vi "Run TCS.vi"(8 "error in (no error)":errorcluster, 11 "AutoExp in":refnum<class "AutoExp.lvclass">) -> (0 "error out":errorcluster, 3 "AutoExp out":refnum<class "AutoExp.lvclass">)   [LabVIEW 2018, in "AutoExp.lvclass"]
uses:
  AutoExp.lvclass
  AutoExp.lvclass/AutoExp.ctl
  State Machine/State Machine.lvclass
  TCS/TCS.lvclass
  Channel/Channel.lvclass
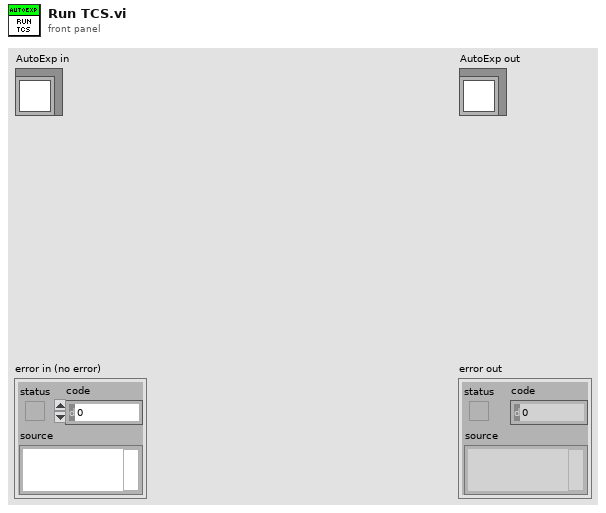
[diagram p1: front panel]
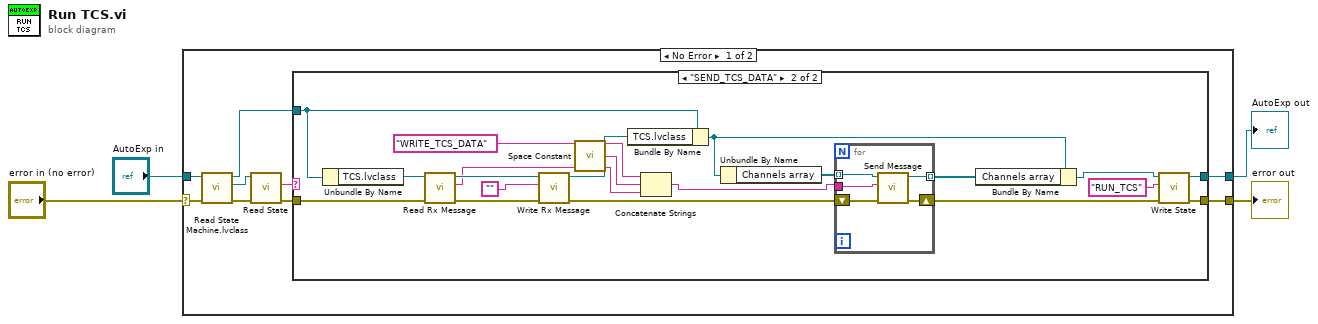
[diagram p0: block diagram]
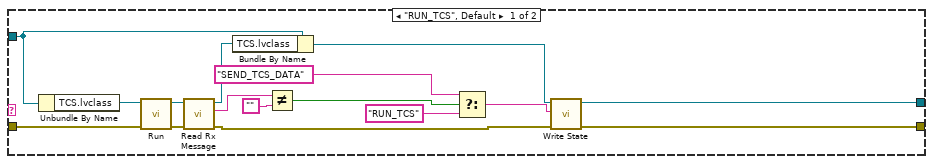
[diagram p2: hidden frame]
diagram:
  n1 = case shown="No Error" "error in (no error)" {
    selector: "error in (no error)" -> [w8 w56]
    tunnel: [w13 w56] -> w3
    tunnel: [w5 w55] -> w1
    tunnel: "AutoExp in" -> [w10 w55]
    frame No Error {
      n2 = call "Read State Machine.lvclass.vi"("error in (no error)"=w8, "AutoExp in"=w10) -> ("error out"=w9:errorcluster, "State Machine.lvclass"=w12:refnum<class "State Machine.lvclass">, "AutoExp out"=w11:refnum<class "AutoExp.lvclass">)  [unwired: 7 in]
      n3 = call-dynamic "Read State.vi"("error in (no error)"=w9, "State Machine in"=w12) -> ("error out"=w6:errorcluster, "State"=w7:string)  [unwired: 7 in, 1 out]
      n4 = case shown="\"SEND_TCS_DATA\"" w7 {
        tunnel: [w25 w36] -> w13
        tunnel: w11 -> [w29 w33]
        tunnel: w6 -> [w14 w34]
        tunnel: [w26 w31] -> w5
        frame "RUN_TCS", Default {
          n5 = Unbundle By Name(w29) -> ("TCS.lvclass"=w17:refnum<class "TCS.lvclass">)
          n6 = call "Run.vi"("error in (no error)"=w14, "TCS in"=w17) -> ("error out"=w15:errorcluster, "TCS out"=w16:refnum<class "TCS.lvclass">)  [unwired: 8 in]
          n7 = call "Read Rx Message.vi"("error in (no error)"=w15, "TCS in"=w16) -> ("error out"=w24:errorcluster, "Rx message"=w23:string, "TCS out"=w28:refnum<class "TCS.lvclass">)  [unwired: 7 in]
          n8 = Bundle By Name(cluster=w29, "TCS.lvclass"=w28) -> (w27:refnum<class "AutoExp.lvclass">)
          n9 = Not Equal?(x=w23, y="") -> (x != y?=w22:bool)
          n10 = Select(t="SEND_TCS_DATA", s=w22, f="RUN_TCS") -> (s? t:f=w19:string)
          n11 = call "Write State.vi"("error in (no error)"=w24, "State"=w19, "AutoExp in"=w27) -> ("error out"=w25:errorcluster, "AutoExp out"=w26:refnum<class "AutoExp.lvclass">)  [unwired: 7 in]
        }
        frame "SEND_TCS_DATA" {
          n12 = Unbundle By Name(w33) -> ("TCS.lvclass"=w35:refnum<class "TCS.lvclass">)
          n13 = call "Read Rx Message.vi"("error in (no error)"=w34, "TCS in"=w35) -> ("error out"=w42:errorcluster, "Rx message"=w40:string, "TCS out"=w41:refnum<class "TCS.lvclass">)  [unwired: 7 in]
          n14 = call "Write Rx Message.vi"("error in (no error)"=w42, "Rx message"="", "TCS in"=w41) -> ("error out"=w46:errorcluster, "TCS out"=w43:refnum<class "TCS.lvclass">)  [unwired: 7 in]
          n15 = call <vilib>:"Space Constant.vi"() -> ("String"=w39:string)
          n16 = Bundle By Name(cluster=w33, "TCS.lvclass"=w43) -> (w47:refnum<class "AutoExp.lvclass">)
          n17 = Concatenate Strings("WRITE_TCS_DATA", w39, w40) -> (w45:string)
          n18 = Unbundle By Name(w47) -> ("Channels array"=w44:refnum<class "Channel.lvclass">[])
          n19 = for {
            tunnel: w44 -> [w50] mode=indexing
            tunnel: [w52] -> w48 mode=indexing
            tunnel: w45 -> [w53]
            shift-right: [w51] -> w49
            shift-left: w46 -> [w54]
            n20 = call "Send Message.vi"("error in (no error)"=w54, "message"=w53, "Channel in"=w50) -> ("error out"=w51:errorcluster, "Channel out"=w52:refnum<class "Channel.lvclass">)  [unwired: 7 in]
          }
          n21 = Bundle By Name(cluster=w47, "Channels array"=w48) -> (w32:refnum<class "AutoExp.lvclass">)
          n22 = call "Write State.vi"("error in (no error)"=w49, "State"="RUN_TCS", "AutoExp in"=w32) -> ("error out"=w36:errorcluster, "AutoExp out"=w31:refnum<class "AutoExp.lvclass">)  [unwired: 7 in]
        }
      }
    }
    frame Error {
    }
  }
  "error out" <- w3
  "AutoExp out" <- w1
